vi "Set BasePath.vi"(8 "error in (no error)":errorcluster, 10 "ErrorLogBasePath":path, 11 "ErrorHandler in":refnum<class "ErrorHandler.lvclass">) -> (0 "error out":errorcluster, 3 "ErrorHandler out":refnum<class "ErrorHandler.lvclass">)   [LabVIEW 2019, in "ErrorHandler.lvclass"]
doc: "Developed by Kevin Thompson\nkevin@thompsonengineering.net\n\nCopyright 2018\nThompson Engineering, LLC"
uses:
  ErrorHandler.lvclass
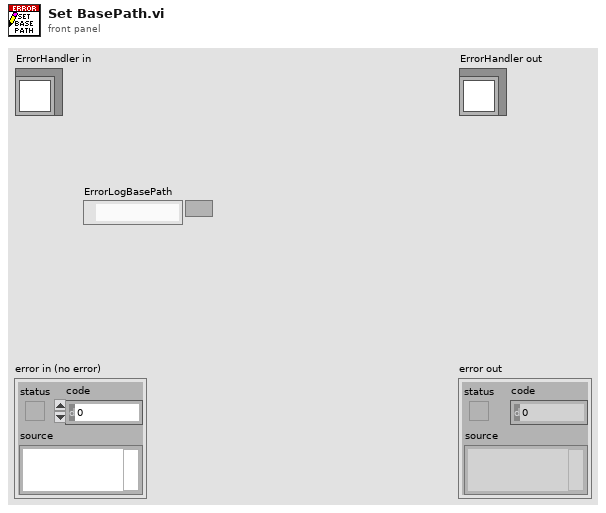
[diagram p1: front panel]
types:
  T1 = typedef "ErrorHandler.lvclass/ObjData--cluster.ctl" = cluster{"AppName":string, "ErrorLogBasePath":path, "ErrorDialogPopUp Disabled":bool, "TerminateAppOnError Enabled":bool, "Public Events":T2, "ErrorList Qref":refnum<queue>}
  T2 = typedef "ErrorHandler.lvclass/Public Events.ctl" = cluster{"ErrorRemote Ev":refnum<user-event>}
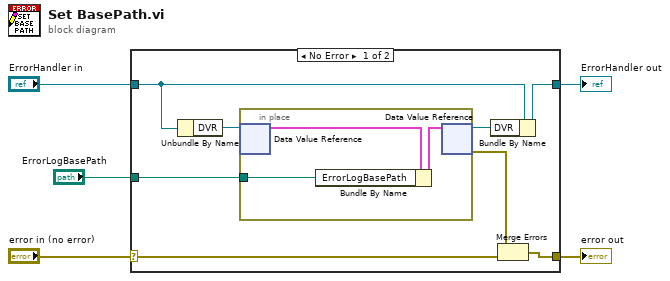
[diagram p0: block diagram]
diagram:
  n1 = case shown="No Error" "error in (no error)" {
    selector: "error in (no error)" -> [w13 w17]
    tunnel: [w9 w17] -> w4
    tunnel: [w11 w18] -> w2
    tunnel: "ErrorHandler in" -> [w10 w18]
    tunnel: "ErrorLogBasePath" -> [w6 _]
    frame No Error {
      n2 = Unbundle By Name(w10) -> ("DVR"=w7:refnum<data-value>)
      n3 = in-place {
        in-place-border: w6 -> [w14]
        n4 = in-place-dvr #1(w7) -> (w16:T1)  [unwired: 1 out]
        n5 = Bundle By Name(cluster=w16, "ErrorLogBasePath"=w14) -> (w15:T1)
        n6 = in-place-dvr #1(w15) -> (w12:refnum<data-value>, w8:errorcluster)
      }
      n7 = Bundle By Name(cluster=w10, "DVR"=w12) -> (w11:refnum<class "ErrorHandler.lvclass">)
      n8 = Merge Errors(w8, w13) -> (w9:errorcluster)
    }
    frame Error {
    }
  }
  "error out" <- w4
  "ErrorHandler out" <- w2
